vi "Create Message Class for Method.vi"(8 "error in (no error)":errorcluster, 9 "Item Refnum":refnum<vi>, 10 "Target":refnum<vi>) -> (0 "error out":errorcluster, 2 "New Send Method":path, 3 "New Class Path":path)   [LabVIEW 2020, in "Message Maker Provider.lvlib"]
uses:
  Message Maker Provider.lvlib
  _Message Maker/_Maker Classes/Coupled Message Scripter/Coupled Message Scripter.lvclass
  _Message Maker/_Maker Classes/Target Method Prototyper/Target Method Prototyper.lvclass
  _Message Maker/_Maker Classes/Message Scripter/Message Scripter.lvclass
  _Message Maker/_Maker Classes/Concrete Send Renamer/Concrete Send Renamer.lvclass
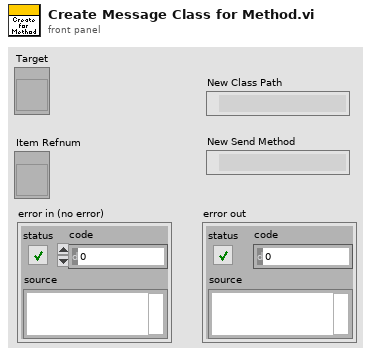
[diagram p1: front panel]
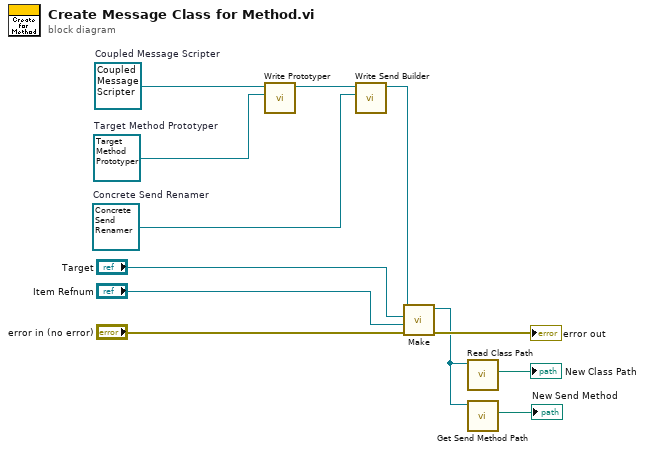
[diagram p0: block diagram]
diagram:
  w4 = refnum<class "Concrete Send Renamer.lvclass"> refnum  # Concrete Send Renamer
  w10 = refnum<class "Target Method Prototyper.lvclass"> refnum  # Target Method Prototyper
  w11 = refnum<class "Coupled Message Scripter.lvclass"> refnum  # Coupled Message Scripter
  n1 = call "Write Prototyper.vi"("Prototyper"=w10, "Message Scripter in"=w11) -> ("Message Scripter out"=w6:refnum<class "Coupled Message Scripter.lvclass">)  [unwired: 9 in]
  n2 = call "Write Send Builder.vi"("Message Maker.lvlib:Send Builder.lvclass"=w4, "Message Scripter in"=w6) -> ("Message Scripter out"=w5:refnum<class "Coupled Message Scripter.lvclass">)  [unwired: 9 in]
  n3 = call-dynamic "Make.vi"("error in (no error)"="error in (no error)", "Item Refnum"="Item Refnum", "Target"="Target", "Coupled Message Scripter"=w5) -> ("error out"=→"error out":errorcluster, "Coupled Message Scripter out"=w9:refnum<class "Coupled Message Scripter.lvclass">)  [unwired: 6 in]
  n4 = call "Read Class Path.vi"("Message Scripter in"=w9) -> ("Class Path"=→"New Class Path":path)  [unwired: 10 in]
  n5 = call "Get Send Method Path.vi"("Message Scripter"=w9) -> ("Send Method Path"=→"New Send Method":path)  [unwired: 10 in]
